vi "Configure Trigger Acquire Source.vi"(8 "error in":errorcluster, 10 "Source":u16(ring) items=["Voltage", "Current", "External", "Bus", "Immediate", "Manual"], 11 "VISA resource name":refnum<visa-resource-name>) -> (0 "error out":errorcluster, 3 "VISA resource name out":refnum<visa-resource-name>)   [LabVIEW 2024, in "IT-M3900C.lvlib"]
doc: "This command sets the trigger source for the Meter function.\n<b>Source</b>\n0: VOLTage\n1: CURRent\n2: EXTernal\n3: BUS\n4: Immediate\n5: Manual"
uses:
  IT-M3900C.lvlib
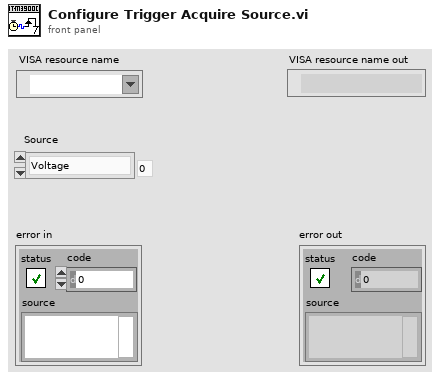
[diagram p1: front panel]
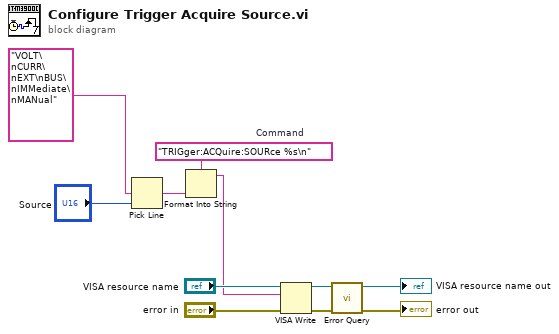
[diagram p0: block diagram]
diagram:
  w5 = "TRIGger:ACQuire:SOURce %s\n"  # Command
  n1 = Pick Line(multi-line string="VOLT\nCURR\nEXT\nBUS\nIMMediate\nMANual", line index="Source") -> (output string=w1:string)  [unwired: 1 in]
  n2 = Format Into String(format string=w5, w1) -> (resulting string=w4:string)  [unwired: 2 in, 1 out]
  n3 = VISA Write(VISA resource name="VISA resource name", write buffer=w4, error in (no error)="error in") -> (VISA resource name out=w8:refnum<visa-resource-name>, error out=w9:errorcluster)  [unwired: 1 out]
  n4 = call "Error Query.vi"("error in"=w9, "VISA resource name"=w8) -> ("error out"=→"error out":errorcluster, "VISA resource name out"=→"VISA resource name out":refnum<visa-resource-name>)  [unwired: 6 in, 2 out]
